vi "Set Speed.vi"(1 "Speed":dbl, 2 "Car.lvclass 2":refnum<class "Car.lvclass">) -> (0 "Car.lvclass":refnum<class "Car.lvclass">)   [LabVIEW 2015, in "Car.lvclass"]
uses:
  Car.lvclass
  Car.lvclass/Car.ctl
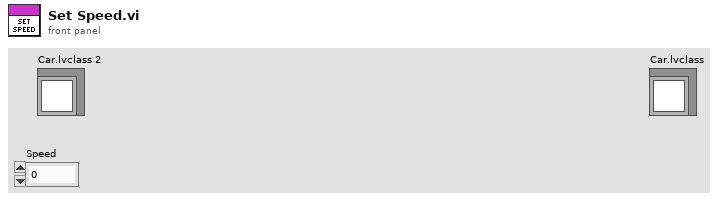
[diagram p1: front panel]
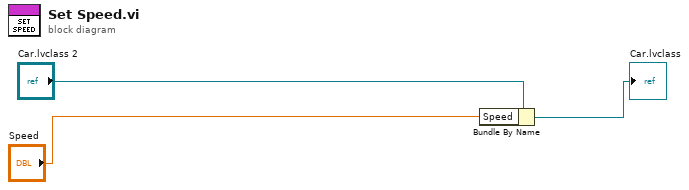
[diagram p0: block diagram]
diagram:
  n1 = Bundle By Name(cluster="Car.lvclass 2", "Speed"="Speed") -> (→"Car.lvclass":refnum<class "Car.lvclass">)
